vi "Close.vi"(8 "error in (no error)":errorcluster, 11 "1553 Component in":refnum<class "1553 Component.lvclass">) -> (0 "error out":errorcluster)   [LabVIEW 2020, in "BCI-1553 API.lvlib" / "1553 Component.lvclass"]
doc: "Closes all the resources allocated by this component. It is strongly suggested to call the 'Clean Up' method before closing a component."
uses:
  1553 Component.lvclass
  1553 Component.lvclass/1553 Component.ctl
  Dependencies/FPGA Interface/FPGA Interface.lvclass
  Dependencies/Virtual Memory Unit/Virtual Memory Unit.lvclass
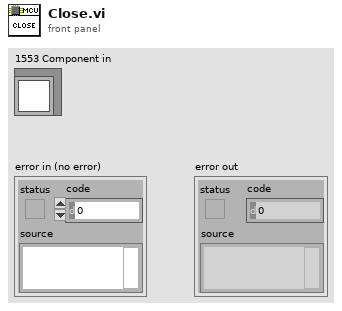
[diagram p1: front panel]
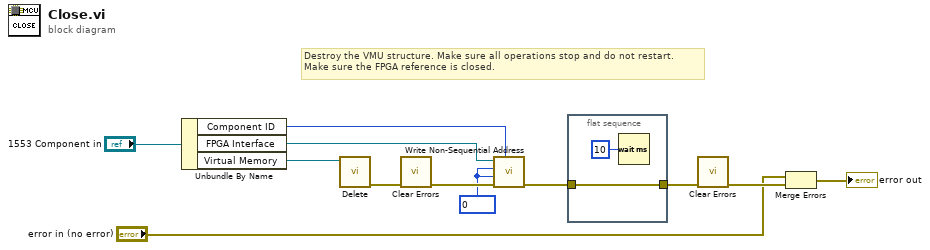
[diagram p0: block diagram]
diagram:
  w6 = u16 0 ("Address")
  # "Destroy the VMU structure. Make sure all operations stop and do not restart.\nMake sure the FPGA reference is closed."
  n1 = Unbundle By Name("1553 Component in") -> ("Component ID"=w3:u8, "FPGA Interface"=w7:refnum<class "FPGA Interface.lvclass">, "Virtual Memory"=w9:refnum<class "Virtual Memory Unit.lvclass">)
  n2 = call "Delete.vi"("Virtual Memory Unit in"=w9) -> ("error out"=w10:errorcluster)  [unwired: 10 in]
  n3 = call <vilib>:"Clear Errors.vi"("error in (no error)"=w10) -> ("error out"=w8:errorcluster)  [unwired: 5 in, 1 out]
  n4 = call-dynamic "Write Non-Sequential Address.vi"("Target IC (1-8)"=w3, "error in (no error)"=w8, "Data"=w6, "Address"=w6, "FPGA Interface in"=w7) -> ("error out"=w5:errorcluster)  [unwired: 6 in]
  n5 = flat-sequence {
    tunnel: [w14] -> w4
    tunnel: w5 -> [w14]
    frame #0 {
      n6 = Wait (ms)(milliseconds to wait=u32 10) -> ()  [unwired: 1 out]
    }
  }
  n7 = call <vilib>:"Clear Errors.vi"("error in (no error)"=w4) -> ("error out"=w12:errorcluster)  [unwired: 5 in, 1 out]
  n8 = Merge Errors("error in (no error)", w12) -> (→"error out":errorcluster)
